vi "MMME P01 SubVI02.vi"(4 "A":bool, 5 "B":bool, 6 "C":bool, 7 "D":bool) -> (0 "W":bool, 1 "X":bool, 2 "Y":bool, 3 "Z":bool)   [LabVIEW 2021]
doc: "El presente programa tiene como finalidad la conversión de número decimal de 0 - 9 a binario considerando los 4 bits \"ABCD\" entregando como salida \"WXYZ\" basándonos en la tabla de verdad que fue propuesta por el profesor.\n- Creador : Mendoza Meza Manuel Everardo\n- Grupo: 3MV5\n- Periodo: 2022/2"
panel:
  # "Mendoza Meza Manuel Everardo"
  # "SUBVI Interno"
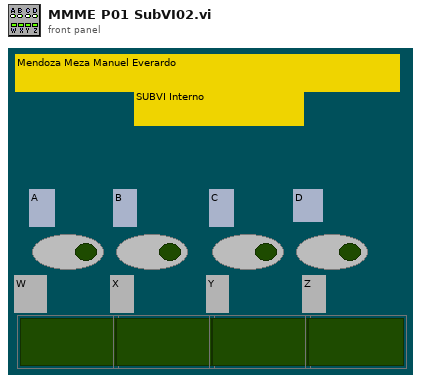
[diagram p1: front panel]
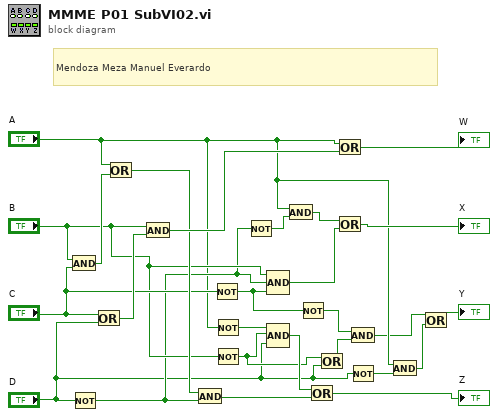
[diagram p0: block diagram]
diagram:
  # "Mendoza Meza Manuel Everardo"
  n1 = And(x="B", y="C") -> (x .and. y?=w23:bool)
  n2 = Not(x="D") -> (.not. x?=w12:bool)
  n3 = Or(x="C", y="D") -> (x .or. y?=w26:bool)
  n4 = Or(x="A", y=w23) -> (x .or. y?=w22:bool)
  n5 = And(x="B", y=w26) -> (x .and. y?=w24:bool)
  n6 = And(x=w22, y=w12) -> (x .and. y?=w20:bool)
  n7 = Not(x="C") -> (.not. x?=w8:bool)
  n8 = Not(x="A") -> (.not. x?=w18:bool)
  n9 = Not(x="B") -> (.not. x?=w11:bool)
  n10 = Not(x=w12) -> (.not. x?=w14:bool)
  n11 = Compound Arithmetic op=AND("B", w12, w8) -> (w9:bool)
  n12 = Compound Arithmetic op=AND(w18, w11, "D") -> (w19:bool)
  n13 = And(x="A", y=w14) -> (x .and. y?=w13:bool)
  n14 = Not(x=w8) -> (.not. x?=w7:bool)
  n15 = Or(x=w19, y=w20) -> (x .or. y?=→"Z":bool)
  n16 = Or(x=w11, y="D") -> (x .or. y?=w10:bool)
  n17 = Or(x="A", y=w24) -> (x .or. y?=→"W":bool)
  n18 = Or(x=w13, y=w9) -> (x .or. y?=→"X":bool)
  n19 = And(x=w7, y=w10) -> (x .and. y?=w1:bool)
  n20 = Not(x="D") -> (.not. x?=w4:bool)
  n21 = And(x="A", y=w4) -> (x .and. y?=w3:bool)
  n22 = Or(x=w1, y=w3) -> (x .or. y?=→"Y":bool)
